vi "READ.vi"() -> (0 "error out":errorcluster, 2 "Result Set":string[][](table) caption="Result Set (from first statement with results)", 3 "appended array":string[][](array[string]))   [LabVIEW 2020, in "Settings.lvlib"]
uses:
  Settings.lvlib
  <vilib>/drjdpowell/SQLite Library/SQL Connection/Open (path).vi
  <vilib>/drjdpowell/SQLite Library/SQL Connection/Open (string).vi
  <vilib>/AdvancedString/Path To Command Line String.vi
  <vilib>/drjdpowell/SQLite Library/SQL Connection/Execute SQL.vi
  <vilib>/drjdpowell/SQLite Library/SQL Connection/Connection.lvclass
  <vilib>/drjdpowell/SQLite Library/SQLite.lvlib
panel:
  in  "error in (no error)":errorcluster
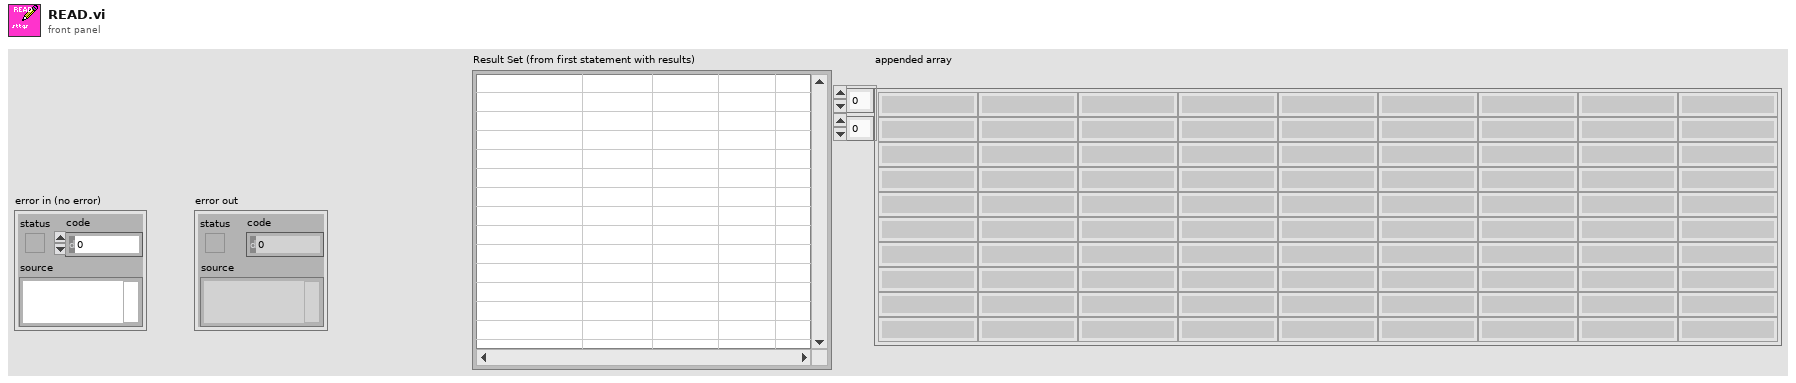
[diagram p1: front panel]
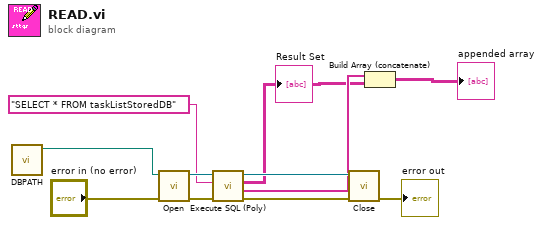
[diagram p0: block diagram]
diagram:
  n1 = call "DBPATH.vi"() -> ("appended path"=w2:path)  [unwired: 11 in]
  n2 = call-poly <vilib>:"Open.vi"("error in (no error)"="error in (no error)", "db file"=w2) -> ("error out"=w11:errorcluster, "SQLite Connection"=w9:refnum<class "Connection.lvclass">)  [unwired: 8 in]
  n3 = call-poly <vilib>:"Execute SQL (Poly).vi"("error in (no error)"=w11, "SQL"="SELECT * FROM taskListStoredDB", "SQLite Connection in"=w9) -> ("error out"=w10:errorcluster, "Column Names"=w4:string[], "Result Set"=w3:string[][], "SQLite Connection"=w8:refnum<class "Connection.lvclass">)  [unwired: 5 in]
  "Result Set" <- w3
  n4 = call-dynamic "Close.vi"("error in (no error)"=w10, "SQLite Connection in"=w8) -> ("error out"=→"error out":errorcluster)  [unwired: 9 in]
  n5 = Build Array (concatenate)(w4, w3) -> (→"appended array":string[][])
